vi "queryBuffer.vi"(8 "error in (no error)":errorcluster, 11 "Electrometer in":refnum<class "Electrometer.lvclass">) -> (0 "error out":errorcluster, 2 "number":i32, 3 "Electrometer out":refnum<class "Electrometer.lvclass">)   [LabVIEW 2016, in "Electrometer.lvclass"]
uses:
  Electrometer.lvclass
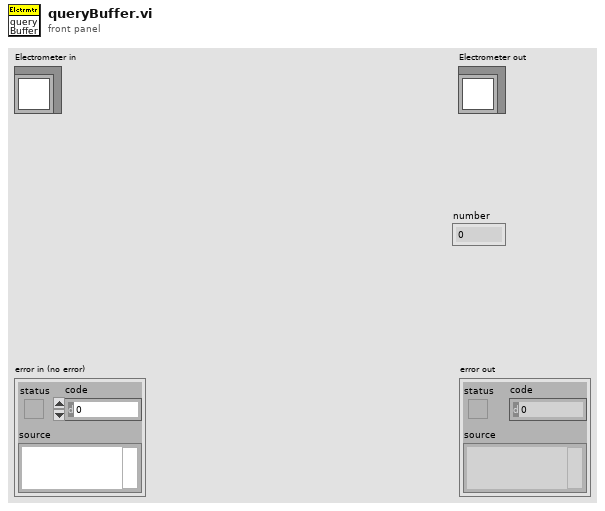
[diagram p1: front panel]
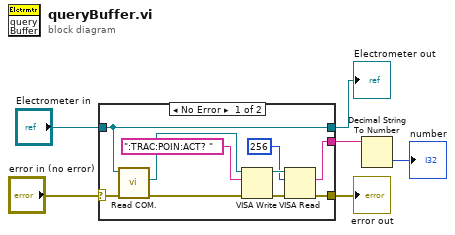
[diagram p0: block diagram]
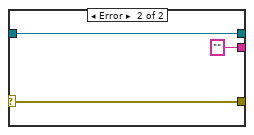
[diagram p2: hidden frame]
diagram:
  n1 = case shown="No Error" "error in (no error)" {
    selector: "error in (no error)" -> [w16 w19]
    tunnel: [w11 w19] -> w3
    tunnel: [w13 w18] -> w5
    tunnel: "Electrometer in" -> [w13 w18]
    tunnel: [w8 "" ("read buffer")] -> w2
    frame No Error {
      n2 = call "Read COM..vi"("error in (no error)"=w16, "Electrometer in"=w13) -> ("error out"=w14:errorcluster, "VISA"=w15:refnum<visa-resource-name>)  [unwired: 7 in, 1 out]
      n3 = VISA Write(VISA resource name=w15, write buffer=":TRAC:POIN:ACT? " ("string"), error in (no error)=w14) -> (VISA resource name out=w10:refnum<visa-resource-name>, error out=w12:errorcluster)  [unwired: 1 out]
      n4 = VISA Read(VISA resource name=w10, byte count=u32 256, error in (no error)=w12) -> (read buffer=w8:string, error out=w11:errorcluster)  [unwired: 2 out]
    }
    frame Error {
    }
  }
  "error out" <- w3
  "Electrometer out" <- w5
  n5 = Decimal String To Number(string=w2) -> (number=→"number":i32)  [unwired: 2 in, 1 out]
